vi "Agilent PWM Set Trigger Source.vi"(7 "Agilent PWM":T1, 8 "error in (no error)":errorcluster, 10 "Trigger Source":T2, 11 "VISA Resource Name":refnum<visa-resource-name>) -> (0 "error out":errorcluster, 3 "dup VISA Resource Name":refnum<visa-resource-name>)   [LabVIEW 2011]
doc: "This VI for the HP 8753 is used to read the sweep type.\n\n0 LINEAR FREQ\n1 LOG FREQ\n2 LIST FREQ\n3 CW TIME\n4 POWER SWEEP"
uses:
  TypeDefs/Agilent PWM Trigger Source.ctl
  TypeDefs/Agilent PWM Instrument Info.ctl
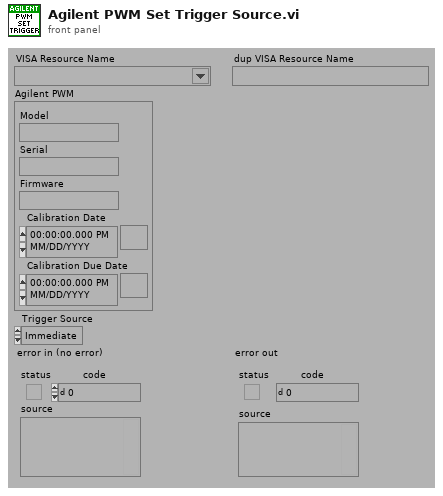
[diagram p1: front panel]
types:
  T1 = typedef "Agilent PWM Instrument Info.ctl" = cluster{"Model":string, "Serial":string, "Firmware":string, "Calibration Date":timestamp, "Calibration Due Date":timestamp}
  T2 = typedef "Agilent PWM Trigger Source.ctl" = enum16{"Immediate", "Bus", "Hold", "Internal", "External"}
  T3 = typedef "Agilent PWM Model.ctl" = enum16{"Not Supported", "E4418X", "E4419X", "U2000X"}
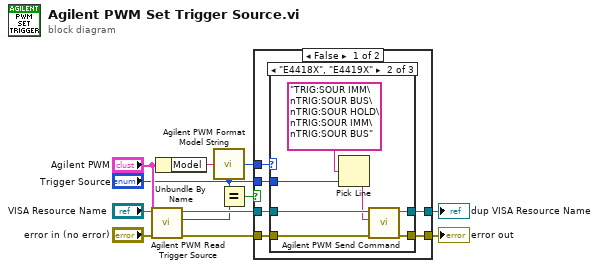
[diagram p0: block diagram]
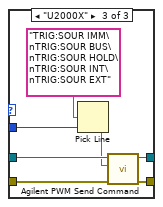
[diagram p3: hidden frame]
diagram:
  n1 = call "Agilent PWM Read Trigger Source.vi"("Agilent PWM"="Agilent PWM", "error in (no error)"="error in (no error)", "VISA Resource Name"="VISA Resource Name") -> ("error out"=w1:errorcluster, "Trigger Source"=w6:T2, "dup VISA Resource Name"=w7:refnum<visa-resource-name>)  [unwired: 6 in]
  n2 = Unbundle By Name("Agilent PWM") -> ("Model"=w10:string)
  n3 = call "Agilent PWM Format Model String.vi"("Model"=w10) -> ("Model"=w3:T3)
  n4 = Equal?(x="Trigger Source", y=w6) -> (x = y?=w5:bool)
  n5 = case shown="False" w5 {
    tunnel: w1 -> [w18 w35]
    tunnel: w7 -> [w17 w36]
    tunnel: [w16 w35] -> w12
    tunnel: [w15 w36] -> w11
    tunnel: "Trigger Source" -> [w14 _]
    tunnel: w3 -> [w13 _]
    frame False {
      n6 = case shown="\"E4418X\", \"E4419X\"" w13 {
        tunnel: w18 -> [w19 w27 w34]
        tunnel: w17 -> [w20 w26 w33]
        tunnel: [w19 w25 w32] -> w16
        tunnel: [w20 w24 w31] -> w15
        tunnel: w14 -> [_ w23 w30]
        frame "Not Supported" {
        }
        frame "E4418X", "E4419X" {
          n7 = Pick Line(multi-line string="TRIG:SOUR IMM\nTRIG:SOUR BUS\nTRIG:SOUR HOLD\nTRIG:SOUR IMM\nTRIG:SOUR BUS" ("write buffer"), line index=w23) -> (output string=w21:string)  [unwired: 1 out]
          n8 = call "Agilent PWM Send Command.vi"("error in (no error)"=w27, "Command"=w21, "VISA Resource Name"=w26) -> ("error out"=w25:errorcluster, "dup VISA Resource Name"=w24:refnum<visa-resource-name>)  [unwired: 2 in, 5 out]
        }
        frame "U2000X" {
          n9 = Pick Line(multi-line string="TRIG:SOUR IMM\nTRIG:SOUR BUS\nTRIG:SOUR HOLD\nTRIG:SOUR INT\nTRIG:SOUR EXT" ("write buffer"), line index=w30) -> (output string=w28:string)  [unwired: 1 out]
          n10 = call "Agilent PWM Send Command.vi"("error in (no error)"=w34, "Command"=w28, "VISA Resource Name"=w33) -> ("error out"=w32:errorcluster, "dup VISA Resource Name"=w31:refnum<visa-resource-name>)  [unwired: 2 in, 5 out]
        }
      }
    }
    frame True {
    }
  }
  "dup VISA Resource Name" <- w11
  "error out" <- w12
